vi "UUTInfomation.vi"(6 "LastUserName":string, 7 "SeqModel?":bool=TRUE, 8 "error in (no error)":errorcluster, 9 "PartNumberData":T1(array[cluster]), 10 "Timeout(ms)":i32, 11 "Sequence Context In":refnum<k7>) -> (0 "error out":errorcluster, 2 "Timeout":bool, 3 "Continue Testing?":bool)   [LabVIEW 2021]
doc: "Custom DUT Information dialog."
uses:
  Data/InitialStates.ctl
  Data/Data.ctl
  <vilib>/addons/TestStand/_TSUtility.llb/TestStand - Set Property Value (Boolean).vi
panel:
  out "Message":string
  in  "Barcode":string
  in  "Cancel":bool
  in  "OK":bool
  in  "Terminate?":bool
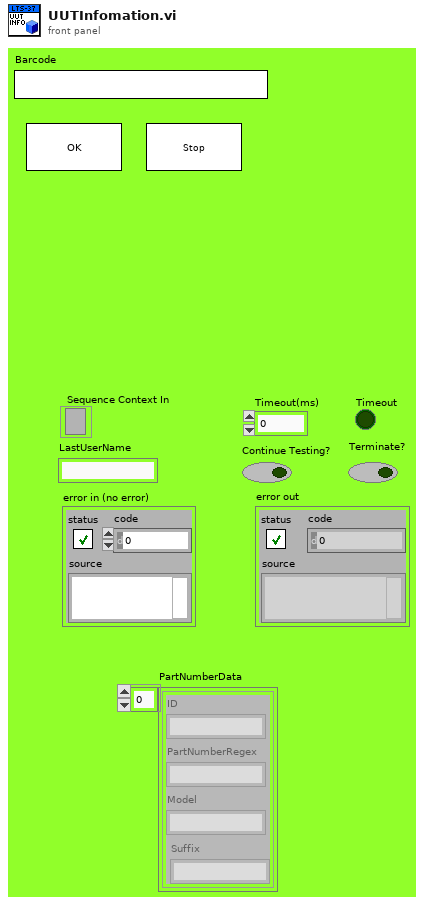
[diagram p1: front panel]
types:
  T1 = cluster{"ID":string, "PartNumberRegex":string, "Model":string, "Suffix":string}[]
  T2 = typedef "Data.ctl" = cluster{"ThisVIref":refnum<vi>, "PnlRef":refnum<vi>, "PartNumberData":cluster{"ID":string, "PartNumberRegex":string, "Model":string, "Suffix":string}[], "Timeout":bool, "ContinueTesting?":bool, "isInitialLogIn":bool, "notifier out":refnum<notifier>}
  T3 = typedef "InitialStates.ctl" = enum16{"Initialize", "Find Regex", "Wait For Event", "Exit"}
  T4 = typedef "TestStand - Status Monitor.ctl" = cluster{"Sequence Context":refnum<k7>, "Execution":refnum<k7>, "Termination Monitor":refnum<k7>}
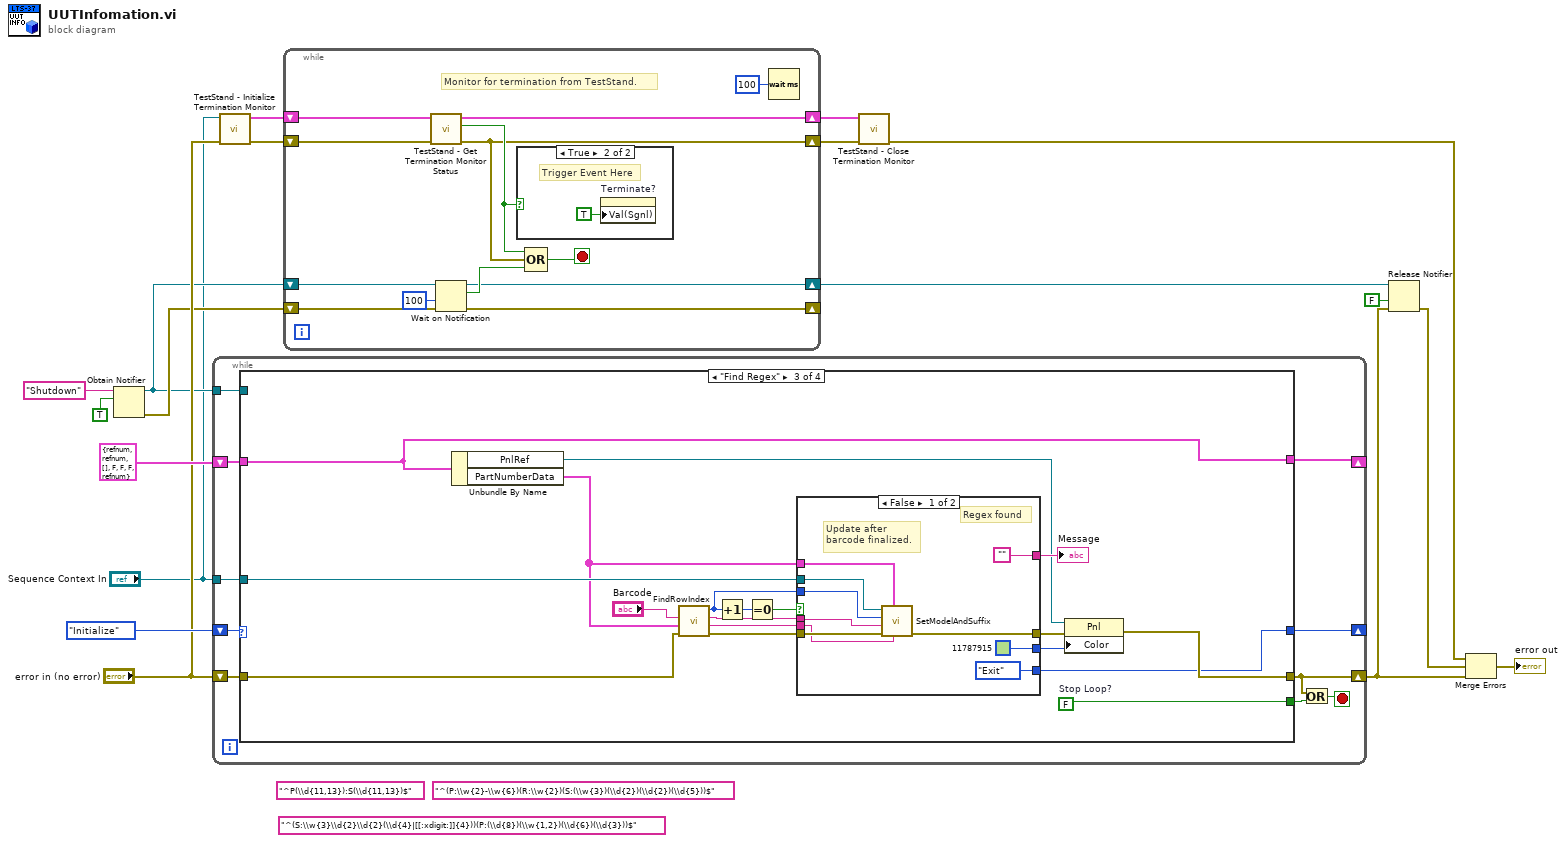
[diagram p0: block diagram]
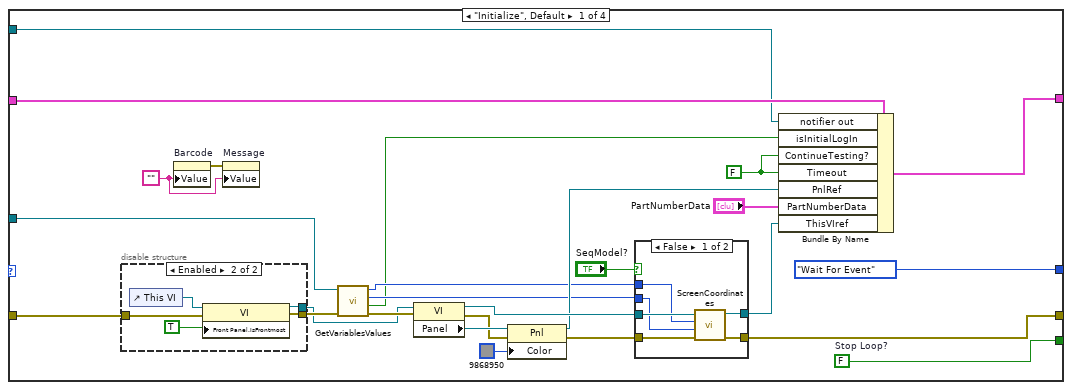
[diagram p3: hidden frame]
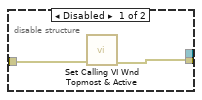
[diagram p4: hidden frame]
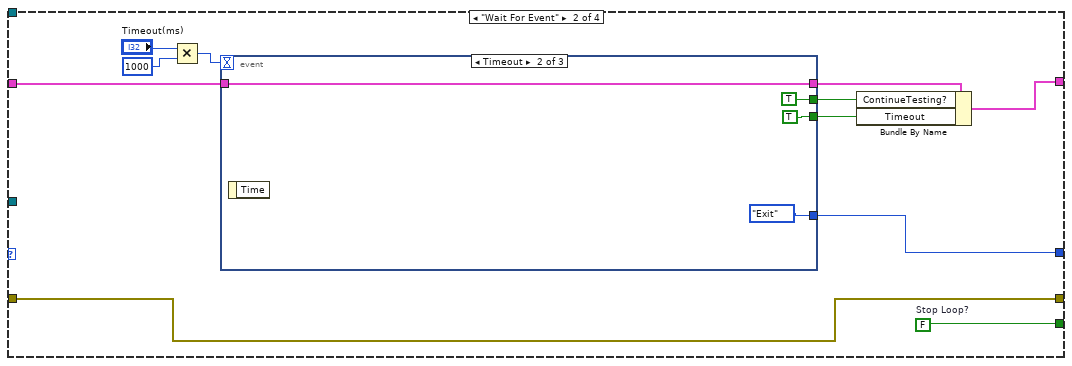
[diagram p6: hidden frame]
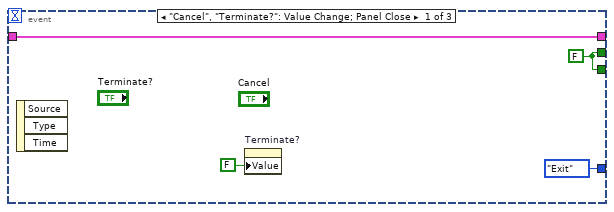
[diagram p7: hidden frame]
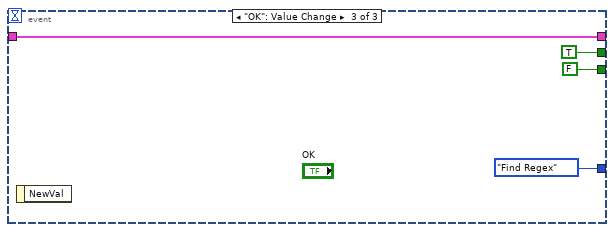
[diagram p8: hidden frame]
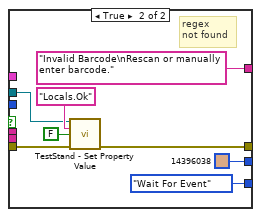
[diagram p9: hidden frame]
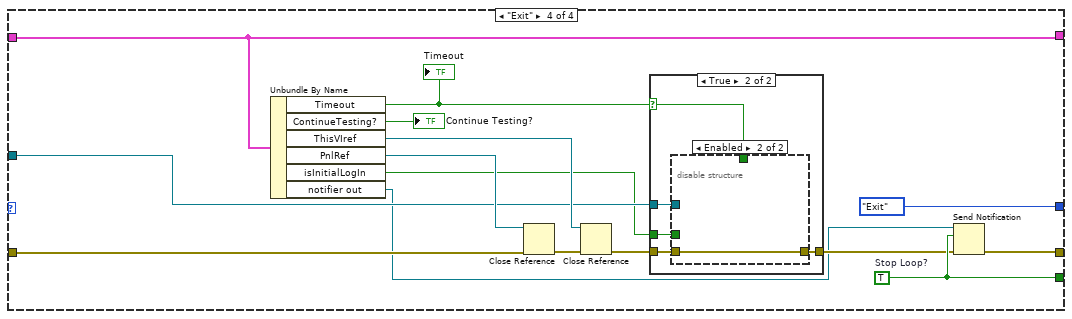
[diagram p10: hidden frame]
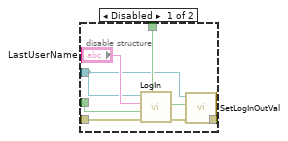
[diagram p12: hidden frame]
diagram:
  (unwired) "^(P:\\w{2}-\\w{6})(R:\\w{2})(S:(\\w{3})(\\d{2})(\\d{2})(\\d{5}))$"
  (unwired) "^(S:\\w{3}\\d{2}\\d{2}(\\d{4}|[[:xdigit:]]{4}))(P:(\\d{8})(\\w{1,2})(\\d{6})(\\d{3}))$"
  (unwired) "^P(\\d{11,13}):S(\\d{11,13})$" ("regular expression")
  n1 = Obtain Notifier(name (unnamed)="Shutdown", notification data type=TRUE) -> (notifier out=w11:refnum<notifier>, error out=w12:errorcluster)  [unwired: 2 in, 1 out]
  n2 = while {
    shift-right: [w23] -> _
    shift-left: InitialStates."Initialize" -> [w28]
    shift-right: [w24] -> _
    shift-left: T2 {"ThisVIref"=refnum, "PnlRef"=refnum, "PartNumberData"=[], "Timeout"=FALSE, "ContinueTesting?"=FALSE, "isInitialLogIn"=FALSE, "notifier out"=refnum} ("Data") -> [w27]
    tunnel: "Sequence Context In" -> [w26]
    shift-right: [w22] -> w2
    shift-left: "error in (no error)" -> [w25]
    tunnel: w11 -> [w19]
    stop <- w20 stop-if-true
    n3 = case shown="\"Find Regex\"" w28 {
      tunnel: w27 -> [w46 w79 w96 w141]
      tunnel: w26 -> [w29 _ w103 w136]
      tunnel: w25 -> [w31 w78 w106 w133]
      tunnel: [w44 w75 w96 w141] -> w24
      tunnel: [InitialStates."Wait For Event" w80 w98 InitialStates."Exit"] -> w23
      tunnel: [w42 w78 w104 w130] -> w22
      tunnel: [w41 w77 w97 w132] -> w21
      tunnel: w19 -> [w30 _ _ _]
      frame "Initialize", Default {
        w36 = FALSE ("Timeout")
        w41 = FALSE  # Stop Loop?
        w50 = ""
        n4 = disable-structure shown="Enabled" {
          disable-tunnel: w31 -> [w56 w60]
          disable-tunnel: [w55 w59] -> w34
          disable-tunnel: [_ w58] -> w32
          frame Disabled {
            n5 = call "Set Calling VI Wnd Topmost & Active.vi"("Error In"=w56) -> ("Error Out"=w55:errorcluster)  [unwired: 10 in]
          }
          frame Enabled {
            n6 = control-ref of="This VI"() -> (w61:refnum<vi>)
            n7 = property class="VI"(reference=w61, error in=w60, "Front Panel.IsFrontmost"=TRUE ("Front Panel Window:Is Frontmost")) -> (reference out=w58:refnum<vi>, error out=w59:errorcluster)
          }
        }
        n8 = property on="Barcode" class="Str"("Value"=w50) -> (error out=w51:errorcluster)  [unwired: 2 in, 1 out]
        n9 = property on="Message" class="Str"(error in=w51, "Value"=w50) -> ()  [unwired: 1 in, 2 out]
        n10 = call "GetVariablesValues.vi"("error in (no error)"=w34, "Sequence Context In"=w29) -> ("error out (no error)"=w33:errorcluster, "isInitialLogIn"=w35:bool, "LeftCoordinates"=w39:i16, "TopCoordinates"=w40:i16)  [unwired: 6 in]
        n11 = property class="VI"(reference=w32, error in=w33) -> (reference out=w48:refnum<vi>, error out=w52:errorcluster, "Panel"=w53:refnum<vi>)
        n12 = property class="Pnl"(reference=w53, error in=w52, "Color"=u32 9868950 ("Color Box")) -> (reference out=w45:refnum<vi>, error out=w49:errorcluster)
        n13 = case shown="False" "SeqModel?" {
          tunnel: w49 -> [w67 w69]
          tunnel: [w66 w69] -> w42
          tunnel: w48 -> [w65 w68]
          tunnel: w40 -> [w64 _]
          tunnel: w39 -> [w63 _]
          tunnel: [w62 w68] -> w37
          frame False {
            n14 = call "ScreenCoordinates.vi"("error in (no error)"=w67, "Left Coordinate"=w63, "Top Coordinate"=w64, "ThisVI"=w65) -> ("error out"=w66:errorcluster, "reference out"=w62:refnum<vi>)  [unwired: 6 in]
          }
          frame True {
          }
        }
        n15 = Bundle By Name(cluster=w46, "notifier out"=w30, "isInitialLogIn"=w35, "ContinueTesting?"=w36, "Timeout"=w36, "PnlRef"=w45, "PartNumberData"="PartNumberData", "ThisVIref"=w37) -> (w44:T2)
      }
      frame "Wait For Event" {
        w77 = FALSE  # Stop Loop?
        n16 = Multiply(x="Timeout(ms)", y=1000) -> (x*y=w72:i32)
        n17 = event shown="[1] Timeout" {
          selector: _ -> [_ _ _]
          dyn-events: _ -> [_ _ _]
          timeout: w72 -> [_ _ _]
          tunnel: [InitialStates."Exit" InitialStates."Exit" InitialStates."Find Regex"] -> w80
          tunnel: [w83 w86 w91] -> w76
          tunnel: w79 -> [w83 w86 w91]
          tunnel: [w82 TRUE TRUE] -> w74
          tunnel: [w82 TRUE ("Timeout") FALSE ("Timeout")] -> w73
          event "Cancel", "Terminate?": Value Change; Panel Close {
            w82 = FALSE
            n18 = event-data() -> ()  [unwired: 1 in, 3 out]
            n19 = property on="Terminate?" class="Bool (strict)"("Value"=FALSE ("Terminate?")) -> ()  [unwired: 2 in, 2 out]
          }
          event Timeout {
            n20 = event-data() -> ()  [unwired: 1 in, 1 out]
          }
          event "OK": Value Change {
            n21 = event-data() -> ()  [unwired: 1 in, 1 out]
          }
        }
        n22 = Bundle By Name(cluster=w76, "ContinueTesting?"=w74, "Timeout"=w73) -> (w75:T2)
      }
      frame "Find Regex" {
        w97 = FALSE  # Stop Loop?
        n23 = Unbundle By Name(w96) -> ("PnlRef"=w107:refnum<vi>, "PartNumberData"=w95:T1)
        n24 = call "FindRowIndex.vi"("error in (no error)"=w106, "PartNumberData"=w95, "Barcode"="Barcode") -> ("error out"=w100:errorcluster, "SerialNumber"=w93:string, "PartNumber"=w94:string, "ArrayIndex"=w102:i32)  [unwired: 4 in, 1 out]
        n25 = Increment(x=w102) -> (x+1=w110:i32)
        n26 = Equal To 0?(x=w110) -> (x = 0?=w109:bool)
        n27 = case shown="False" w109 {
          tunnel: ["" "Invalid Barcode\nRescan or manually enter barcode." ("message")] -> w108
          tunnel: [u32 11787915 ("Color Box") u32 14396038 ("Color Box")] -> w105
          tunnel: w103 -> [w116 w122]
          tunnel: w102 -> [w115 _]
          tunnel: w95 -> [w113 _]
          tunnel: w100 -> [w118 w123]
          tunnel: [w117 w121] -> w99
          tunnel: [InitialStates."Exit" InitialStates."Wait For Event"] -> w98
          tunnel: w94 -> [w112 _]
          tunnel: w93 -> [w111 _]
          frame False {
            # "Update after\nbarcode finalized."
            # "Regex found"
            n28 = call "SetModelAndSuffix.vi"("Serial Number"=w111, "PartNumberData"=w113, "error in (no error)"=w118, "Part Number"=w112, "ArrayIndex"=w115, "Sequence Context In"=w116) -> ("error out"=w117:errorcluster)  [unwired: 4 in, 1 out]
          }
          frame True {
            # "regex \nnot found"
            n29 = call-poly <vilib>:"TestStand - Set Property Value.vi"("Sequence Context In"=w122, "Lookup String"="Locals.Ok", "New Value"=FALSE, "error in (no error)"=w123) -> ("error out"=w121:errorcluster)  [unwired: 10 in, 1 out]
          }
        }
        "Message" <- w108
        n30 = property class="Pnl"(reference=w107, error in=w99, "Color"=w105) -> (error out=w104:errorcluster)  [unwired: 1 out]
      }
      frame "Exit" {
        w132 = TRUE  # Stop Loop?
        n31 = Unbundle By Name(w141) -> ("Timeout"=w137:bool, "ContinueTesting?"=→"Continue Testing?":bool, "ThisVIref"=w139:refnum<vi>, "PnlRef"=w140:refnum<vi>, "isInitialLogIn"=w134:bool, "notifier out"=w129:refnum<notifier>)
        "Timeout" <- w137
        n32 = Close Reference(reference=w140, error in (no error)=w133) -> (error out=w142:errorcluster)
        n33 = Close Reference(reference=w139, error in (no error)=w142) -> (error out=w135:errorcluster)
        n34 = case shown="True" w137 {
          selector: w137 -> [_ w148]
          tunnel: w136 -> [_ w145]
          tunnel: w135 -> [w144 w149]
          tunnel: [w144 w146] -> w131
          tunnel: w134 -> [_ w147]
          frame False {
          }
          frame True {
            n35 = disable-structure shown="Enabled" {
              disable-tunnel: w149 -> [w157 w158]
              disable-tunnel: w148 -> [w156 _]
              disable-tunnel: w147 -> [w155 _]
              disable-tunnel: [w152 w158] -> w146
              disable-tunnel: w145 -> [w151 _]
              frame Disabled {
                n36 = call "LogIn.vi"("Timeout"=w156, "error in (no error)"=w157, "IsInitialLogin"=w155, "LastUserName"="LastUserName", "Sequence Context In"=w151) -> ("error out"=w153:errorcluster, "logOut"=w150:bool)  [unwired: 4 in, 1 out]
                n37 = call "SetLogInOutVal.vi"("error in (no error)"=w153, "logOut"=w150, "Sequence Context In"=w151) -> ("error out"=w152:errorcluster)  [unwired: 8 in]
              }
              frame Enabled {
              }
            }
          }
        }
        n38 = Send Notification(notification=w132, notifier=w129, error in (no error)=w131) -> (error out=w130:errorcluster)  [unwired: 1 out]
      }
    }
    n39 = Or(x=w22, y=w21) -> (x .or. y?=w20:bool)
  }
  n40 = call <vilib>:"TestStand - Initialize Termination Monitor.vi"("error in (no error)"="error in (no error)", "Sequence Context In"="Sequence Context In") -> ("error out"=w5:errorcluster, "Status Monitor Out"=w7:T4)  [unwired: 8 in]
  n41 = while {
    shift-right: [w170] -> w6
    shift-left: w7 -> [w171]
    shift-right: [w166] -> w4
    shift-left: w5 -> [w169]
    shift-right: [w162] -> w8
    shift-left: w11 -> [w163]
    shift-right: [w160] -> _
    shift-left: w12 -> [w161]
    stop <- w165 stop-if-true
    # "Monitor for termination from TestStand."
    n42 = call <vilib>:"TestStand - Get Termination Monitor Status.vi"("error in (no error)"=w169, "Status Monitor In"=w171) -> ("error out"=w166:errorcluster, "Terminating or Aborting"=w167:bool, "Status Monitor Out"=w170:T4)  [unwired: 7 in]
    n43 = Wait on Notification(notifier=w163, timeout in ms (-1)=100, error in (no error)=w161) -> (notifier out=w162:refnum<notifier>, notification=w164:bool, error out=w160:errorcluster)  [unwired: 1 in, 1 out]
    n44 = case shown="True" w167 {
      frame False {
      }
      frame True {
        # "Trigger Event Here"
        n45 = property on="Terminate?" class="Bool (strict)"("Val(Sgnl)"=TRUE ("Value (Signaling)")) -> ()  [unwired: 2 in, 2 out]
      }
    }
    n46 = Compound Arithmetic op=OR(w167, w166, w164) -> (w165:bool)
    n47 = Wait (ms)(milliseconds to wait=u32 100) -> ()  [unwired: 1 out]
  }
  n48 = call <vilib>:"TestStand - Close Termination Monitor.vi"("error in (no error)"=w4, "Status Monitor In"=w6) -> ("error out"=w10:errorcluster)  [unwired: 9 in]
  n49 = Release Notifier(notifier=w8, force destroy? (F)=FALSE, error in (no error)=w2) -> (error out=w9:errorcluster)  [unwired: 2 out]
  n50 = Merge Errors(w10, w9, w2) -> (→"error out":errorcluster)
